vi "cv_01-01_GenerateDisplay.vi"() -> ()   [LabVIEW 2013]
doc: "Use this template to simulate the generation and display of data.\nNote: LabVIEW enables automatic error handling by default for VIs you create from this template."
uses:
  Instance           1 27Saved   GenerateDisplay.vit .vi
panel:
  in  "Knob":dbl(knob) scale=0.0..5.0
  out "Waveform Graph":dynamicdata(graph)
  in  "stop":bool
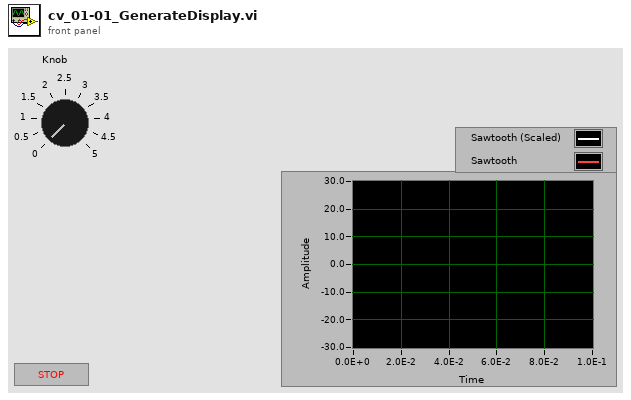
[diagram p1: front panel]
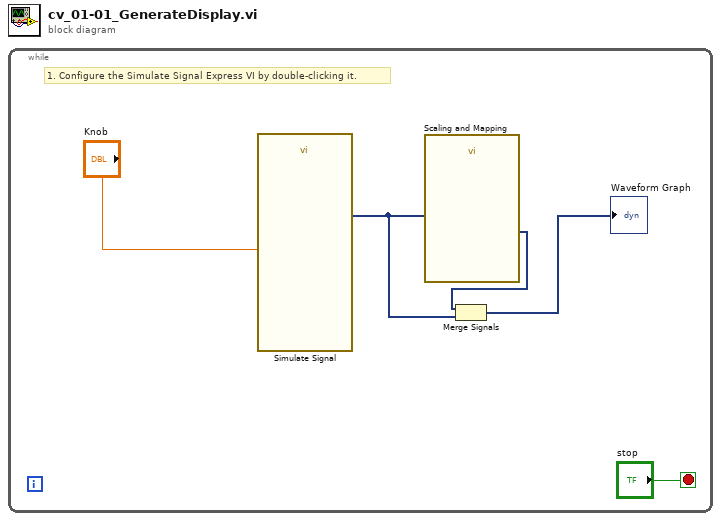
[diagram p0: block diagram]
diagram:
  n1 = while {
    stop <- "stop" stop-if-true
    # "1. Configure the Simulate Signal Express VI by double-clicking it."
    n2 = call "Simulate Signal"("Amplitude"="Knob") -> ("Sawtooth"=w1:dynamicdata)  [unwired: 13 in, 1 out]
    n3 = call "Scaling and Mapping"("Signals"=w1) -> ("Scaled Signals"=w2:dynamicdata)  [unwired: 9 in, 1 out]
    n4 = Merge Signals(w2, w1) -> (→"Waveform Graph":dynamicdata)
  }
